vi "Transmission-octet.vi"() -> ()   [LabVIEW 2019]
uses:
  <vilib>/rvi/eio/common/nirviEmuTemplateMethod_errors.vi
  <vilib>/eio/EIONode/EIONode.xnode
panel:
  in  "DATA":i16[](array[numeric])
  out "DATA + ACK":i16[](array[numeric])
  out "element":i16
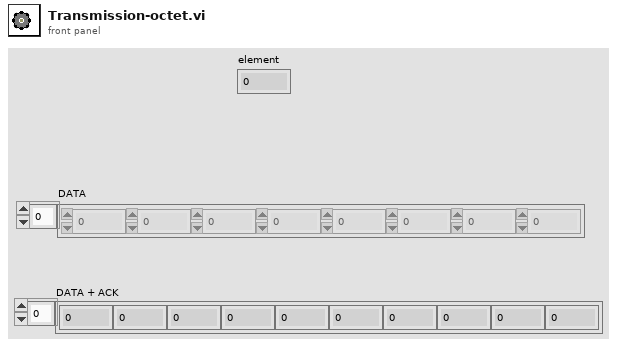
[diagram p1: front panel]
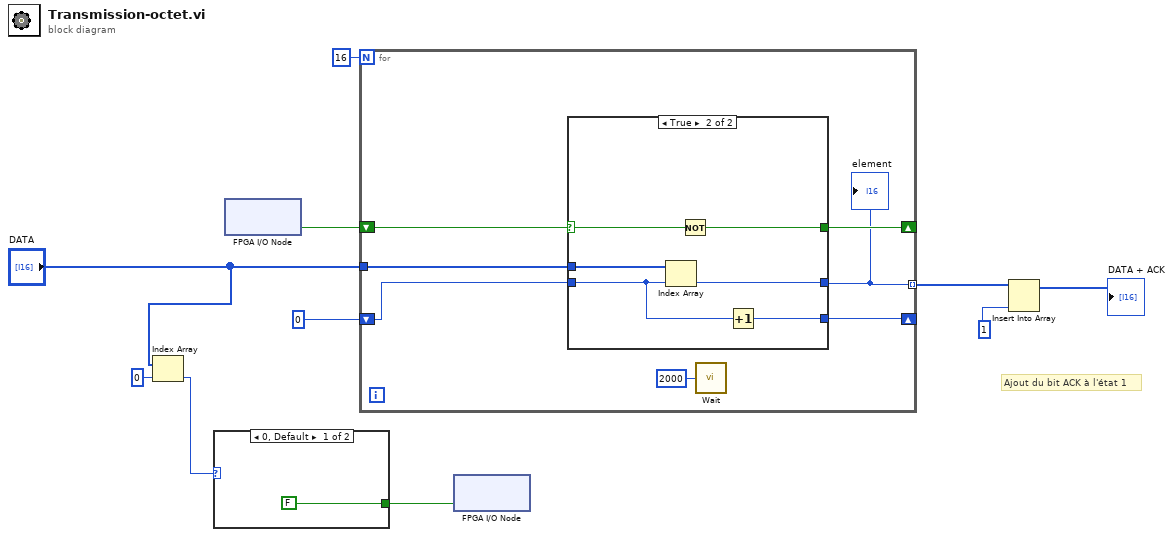
[diagram p0: block diagram]
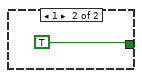
[diagram p2: hidden frame]
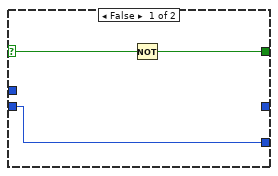
[diagram p3: hidden frame]
diagram:
  # "Ajout du bit ACK à l'état 1"
  n1 = Index Array(array="DATA", index=0) -> (element=w3:i16)
  n2 = case shown="0, Default" w3 {
    tunnel: [FALSE ("SDA") TRUE] -> w2
    frame 0, Default {
    }
    frame 1 {
    }
  }
  n3 = xnode "FPGA I/O Node"() -> ("SCL"=w9:bool)  [unwired: 1 in, 1 out]
  n4 = for {
    N: 16 -> [_]
    tunnel: "DATA" -> [w19]
    shift-right: [w17] -> _
    shift-left: w9 -> [w18]
    shift-right: [w15] -> _
    shift-left: i16 0 -> [w16]
    tunnel: [w13] -> w7 mode=indexing
    n5 = case shown="True" w18 {
      selector: w18 -> [w22 w27]
      tunnel: w19 -> [_ w28]
      tunnel: [w21 w26] -> w17
      tunnel: w16 -> [w20 w25]
      tunnel: [w20 w24] -> w15
      tunnel: [_ w23] -> w13
      frame False {
        n6 = Not(x=w22) -> (.not. x?=w21:bool)
      }
      frame True {
        n7 = Index Array(array=w28, index=w25) -> (element=w23:i16)
        n8 = Not(x=w27) -> (.not. x?=w26:bool)
        n9 = Increment(x=w25) -> (x+1=w24:i16)
      }
    }
    "element" <- w13
    n10 = call "Wait"("Count(mSec)"=u32 2000) -> ()  [unwired: 1 out]
  }
  n11 = xnode "FPGA I/O Node"("SDA"=w2) -> ()  [unwired: 1 in, 1 out]
  n12 = Insert Into Array(array=w7, new element=i16 1) -> (→"DATA + ACK":i16[])  [unwired: 1 in]
